vi "Solve2.vi"(8 "Error In":errorcluster, 11 "object in":refnum<class "2021_1.lvclass">) -> (0 "Error Out":errorcluster, 2 "Result":u64, 3 "object out":refnum<class "2021_1.lvclass">)   [LabVIEW 2020, in "2021_1.lvclass"]
uses:
  2021_1.lvclass
  2021_1.lvclass/2021_1.ctl
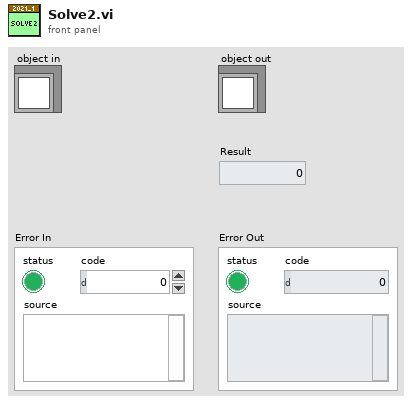
[diagram p1: front panel]
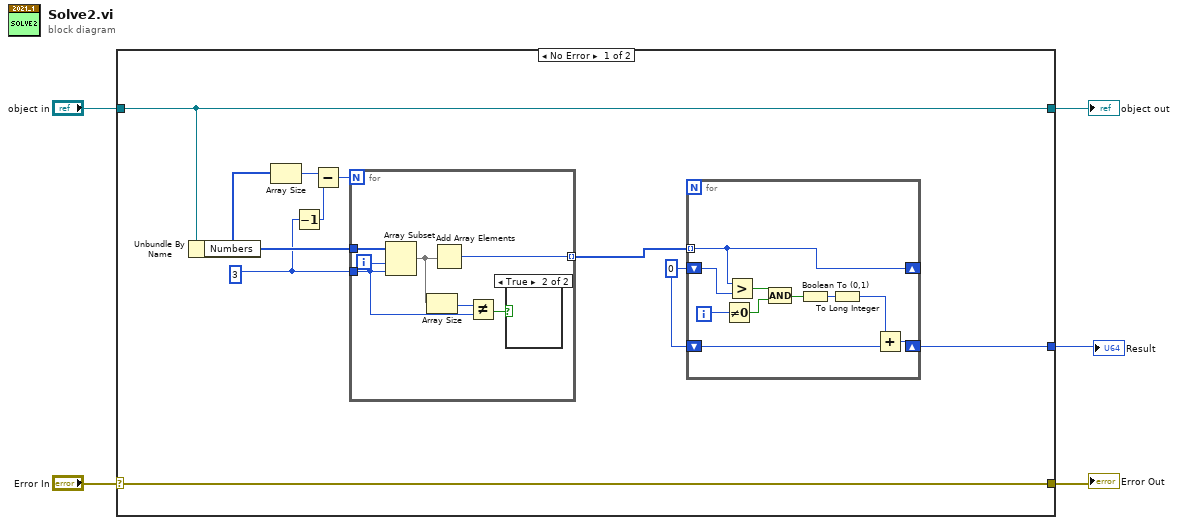
[diagram p0: block diagram]
diagram:
  n1 = case shown="No Error" "Error In" {
    selector: "Error In" -> [w15 w34]
    tunnel: [w15 w34] -> w4
    tunnel: [w14 w33] -> w2
    tunnel: "object in" -> [w14 w33]
    tunnel: [w12 _] -> w1
    frame No Error {
      w8 = 3 ("y")
      w13 = 0
      n2 = Unbundle By Name(w14) -> ("Numbers"=w9:i32[])
      n3 = Array Size(array=w9) -> (size(s)=w11:i32)
      n4 = Decrement(x=w8) -> (x-1=w7:i32)
      n5 = Subtract(x=w11, y=w7) -> (x-y=w10:i32)
      n6 = for {
        N: w10 -> [_]
        tunnel: w9 -> [w22]
        tunnel: w8 -> [w18]
        tunnel: [w16] -> w6 mode=indexing
        i -> [w21]
        n7 = Array Subset(array=w22, index=w21, length=w18) -> (w20:i32[])
        n8 = Array Size(array=w20) -> (size(s)=w19:i32)
        n9 = Add Array Elements(numeric array=w20) -> (sum=w16:i32)
        n10 = Not Equal?(x=w19, y=w18) -> (x != y?=w17:bool)
        n11 = case shown="True" w17 {
          frame False {
          }
          frame True {
          }
        }
      }
      n12 = for {
        tunnel: w6 -> [w32] mode=indexing
        shift-right: [w32] -> _
        shift-left: w13 -> [w31]
        shift-right: [w24] -> w12
        shift-left: w13 -> [w25]
        i -> [w28]
        n13 = Not Equal To 0?(x=w28) -> (x != 0?=w29:bool)
        n14 = Greater?(x=w32, y=w31) -> (0:w30:bool)
        n15 = Compound Arithmetic op=AND(w30, w29) -> (w27:bool)
        n16 = Boolean To (0,1)(Boolean=w27) -> (0, 1=w26:i16)
        n17 = To Long Integer(number=w26) -> (32bit integer=w23:i32)
        n18 = Add(x=w23, y=w25) -> (x+y=w24:i32)
      }
    }
    frame Error {
    }
  }
  "Error Out" <- w4
  "object out" <- w2
  "Result" <- w1
